vi "000AH_电导率_温度补偿系数写入.vi"(8 "error in (no error)":errorcluster caption="错误输入（无错误）", 10 "数值":sgl, 11 "MB_Serial session in":refnum<class "MB_Master_Serial.lvclass">) -> (0 "error out":errorcluster caption="错误输出", 3 "MB_Serial session out":refnum<class "MB_Master_Serial.lvclass">)   [LabVIEW 2016, in "国弘多参数.lvlib"]
uses:
  <vilib>/Plasmionique/MB Master/MB_Master_Serial/MB_Master_Serial.lvclass
  C:/Program Files (x86)/National Instruments/LabVIEW 2016/vi.lib/Plasmionique/MB Master/MB_Master/MB_Master.lvclass
  <vilib>/Plasmionique/MB Master/MB Master.lvlib
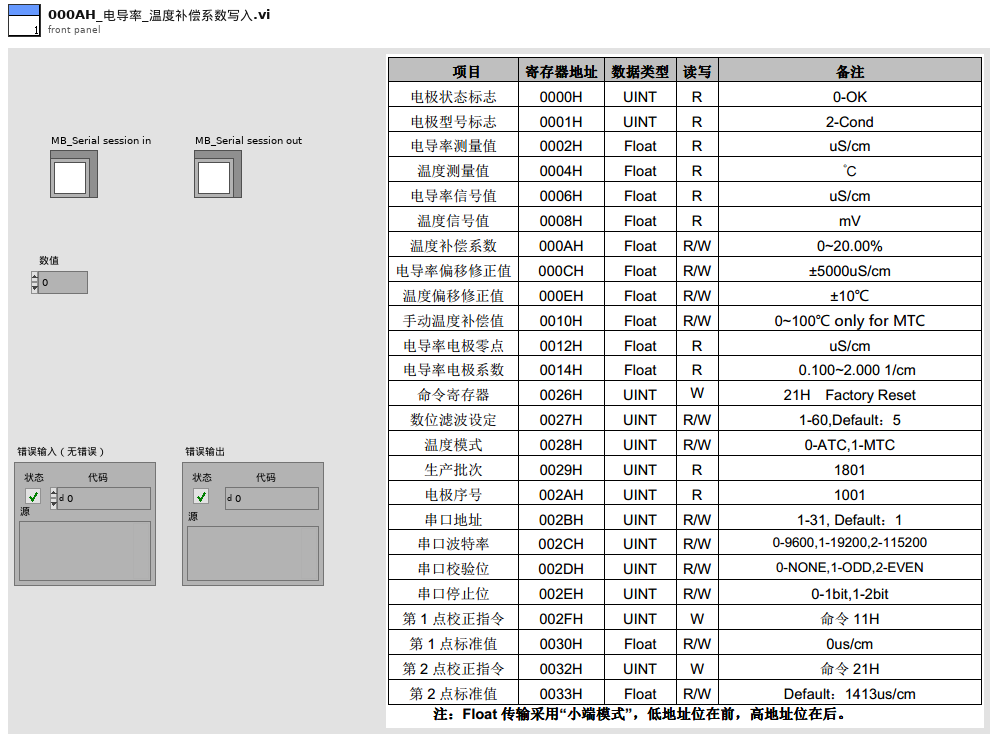
[diagram p1: front panel]
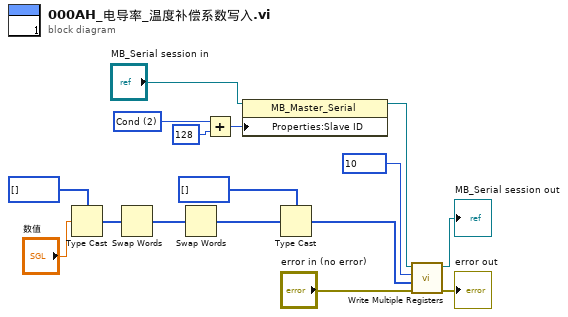
[diagram p0: block diagram]
diagram:
  w9 = u16 2 items=["NULL", "pH", "Cond", "DO", "Turb"] ("数值")
  n1 = Type Cast(type=u32[] [] ("数组 2"), x="数值") -> (*(type *) &x=w10:u32[])
  n2 = Swap Words(1:w10) -> (0:w2:u32[])
  n3 = Swap Words(1:w2) -> (0:w3:u32[])
  n4 = Add(x=w9, y=u16 128) -> (x+y=w8:u16)
  n5 = property class="MB_Master_Serial"(reference="MB_Serial session in", "Properties:Slave ID"=w8) -> (reference out=w5:refnum<class "MB_Master_Serial.lvclass">)  [unwired: 1 in, 1 out]
  n6 = Type Cast(type=u16[] [] ("数组 2"), x=w3) -> (*(type *) &x=w1:u16[])
  n7 = call <vilib>:"Write Multiple Registers.vi"("error in (no error)"="error in (no error)", "values"=w1, "starting address"=u16 10, "MB session in"=w5) -> ("error out"=→"error out":errorcluster, "MB session out"=→"MB_Serial session out":refnum<class "MB_Master_Serial.lvclass">)  [unwired: 6 in]
